vi "Make MD5 from string.vi"(11 "String":string) -> (3 "MD5 message-digest":string)   [LabVIEW 2010]
panel:
  out "error out":errorcluster
  in  "error in (no error)":errorcluster
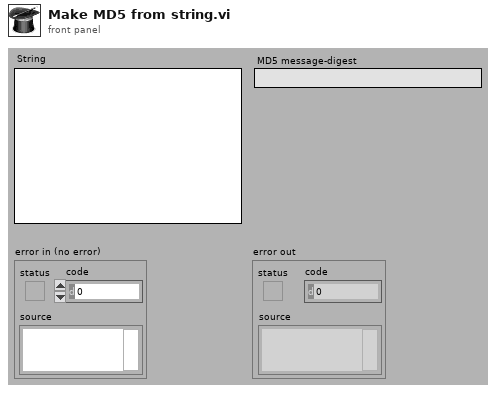
[diagram p1: front panel]
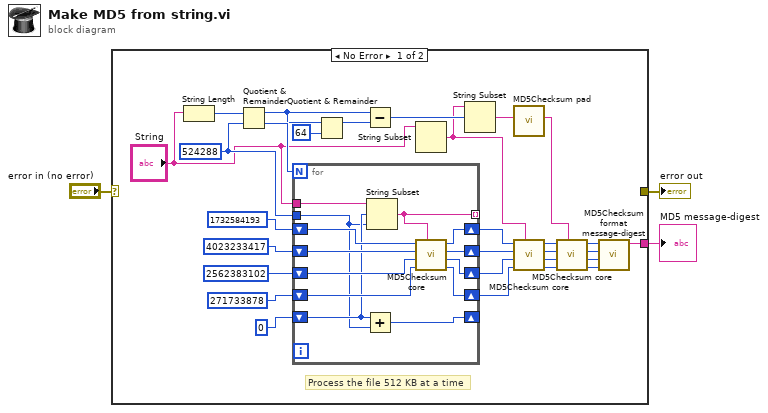
[diagram p0: block diagram]
diagram:
  n1 = case shown="No Error" "error in (no error)" {
    selector: "error in (no error)" -> [_ w46]
    tunnel: [_ w46] -> w3
    tunnel: [w23 _] -> w1
    frame No Error {
      w22 = 524288 ("y")
      # "Process the file 512 KB at a time"
      n2 = String Length(string="String") -> (length=w21:i32)
      n3 = Quotient & Remainder(x=w21, y=w22) -> (x-y*floor(x/y)=w4:i32, floor(x/y)=w20:i32)
      n4 = for {
        N: w20 -> [_]
        shift-right: [w35] -> _
        shift-left: i64 0 ("offset") -> [w36]
        shift-right: [w45] -> w27
        shift-left: u32 1732584193 ("s1") -> [w41]
        shift-right: [w44] -> w26
        shift-left: u32 4023233417 ("s2") -> [w40]
        shift-right: [w43] -> w25
        shift-left: u32 2562383102 ("s3") -> [w39]
        shift-right: [w42] -> w24
        shift-left: u32 271733878 ("s4") -> [w38]
        tunnel: "String" -> [w37]
        tunnel: w22 -> [w34]
        tunnel: [w33] -> _ mode=indexing
        n5 = Add(x=w36, y=w34) -> (x+y=w35:i64)
        n6 = String Subset(string=w37, offset (0)=w36, length (rest)=w34) -> (substring=w33:string)
        n7 = call <vilib>:"MD5Checksum core.vi"("Input String"=w33, "s4 in"=w38, "s3 in"=w39, "s2 in"=w40, "s1 in"=w41) -> ("s4 out"=w42:u32, "s3 out"=w43:u32, "s2 out"=w44:u32, "s1 out"=w45:u32)  [unwired: 3 in]
      }
      n8 = Quotient & Remainder(x=w4, y=64) -> (x-y*floor(x/y)=w17:i32)  [unwired: 1 out]
      n9 = Subtract(x=w4, y=w17) -> (x-y=w18:i32)
      n10 = String Subset(string="String") -> (substring=w6:string)  [unwired: 2 in]
      n11 = String Subset(string=w6, offset (0)=w18) -> (substring=w19:string)  [unwired: 1 in]
      n12 = call <vilib>:"MD5Checksum pad.vi"("Last Part of Message String"=w19) -> ("Padding"=w5:string)  [unwired: 10 in]
      n13 = call <vilib>:"MD5Checksum core.vi"("Input String"=w6, "s4 in"=w24, "s3 in"=w25, "s2 in"=w26, "s1 in"=w27) -> ("s4 out"=w10:u32, "s3 out"=w11:u32, "s2 out"=w12:u32, "s1 out"=w14:u32)  [unwired: 3 in]
      n14 = call <vilib>:"MD5Checksum core.vi"("Input String"=w5, "s4 in"=w10, "s3 in"=w11, "s2 in"=w12, "s1 in"=w14) -> ("s4 out"=w7:u32, "s3 out"=w8:u32, "s2 out"=w9:u32, "s1 out"=w13:u32)  [unwired: 3 in]
      n15 = call <vilib>:"MD5Checksum format message-digest.vi"("s4"=w7, "s3"=w8, "s2"=w9, "s1"=w13) -> ("MD5 message-digest"=w23:string)  [unwired: 7 in]
    }
    frame Error {
    }
  }
  "error out" <- w3
  "MD5 message-digest" <- w1
